vi "test Get-Set-Get Parameter Definitions.vi"(8 "error in":errorcluster, 11 "TestCase in":refnum<class "Scripting.lvclass">) -> (0 "error out":errorcluster, 3 "TestCase out":refnum<class "Scripting.lvclass">)   [LabVIEW 2020, in "Scripting.lvclass"]
uses:
  Scripting.lvclass
  Shared/Parameter Definition.ctl
  <vilib>/NI/NI VeriStand Encoding and Decoding/Encoding.ctl
  Shared/Direction.ctl
  Shared/SDI.ctl
  Shared/Transfer Type.ctl
  Scripting.lvclass/Scripting.ctl
  <vilib>/addons/_JKI Toolkits/VI Tester/TestCase.llb/TestCase.lvclass
  Scripting/AIM/AIM ARINC 429 Scripting.lvlib
  <vilib>/NI/NI VeriStand Encoding and Decoding/Encoding and Decoding.lvlib
  Shared/Transfer Speed.ctl
  C:/Program Files (x86)/National Instruments/LabVIEW 2020/vi.lib/addons/_JKI Toolkits/VI Tester/TestCase.llb/TestCase.lvclass
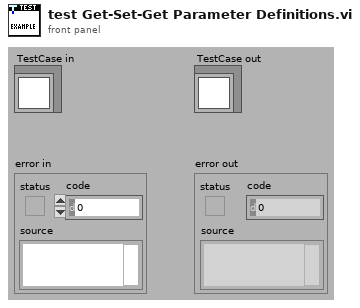
[diagram p1: front panel]
types:
  T1 = typedef "Transfer Speed.ctl" = enum16{"LO (12.5 kb/s)", "HI (100 kb/s)"}
  T2 = typedef "Transfer Type.ctl" = enum16{"Scheduled", "Acyclic", "Block", "Strobe"}
  T3 = typedef "Direction.ctl" = enum16{"Rx", "Tx"}
  T4 = typedef "SDI.ctl" = i32
  T5 = typedef "Parameter Definition.ctl" = cluster{"start index":i32, "size":i32, "encoding":T6, "signed":bool, "scale multiplier":dbl, "scale offset":dbl, "default value":dbl}
  T6 = typedef "Encoding and Decoding.lvlib/Encoding.ctl" = enum16{"BNR", "BCD", "Discrete"}
  T7 = typedef "Custom Device API.lvlib/Custom Device Item Ref.ctl" = u64
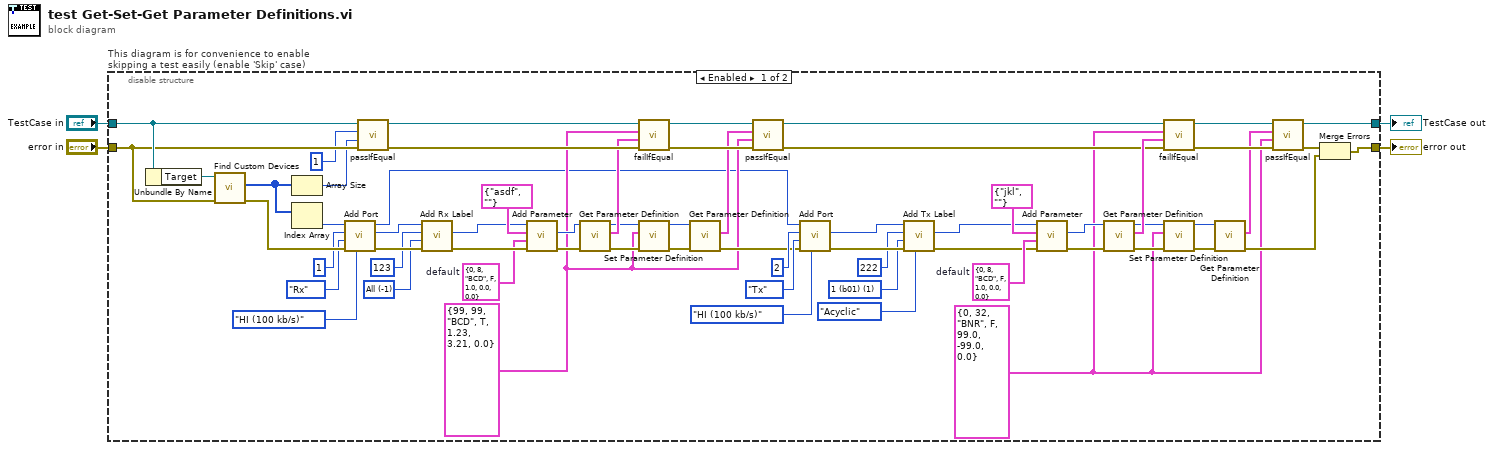
[diagram p0: block diagram]
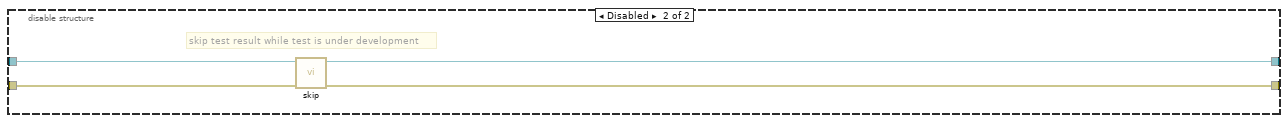
[diagram p2: hidden frame]
diagram:
  n1 = disable-structure "This diagram is for convenience to enable skipping a test easily (enable 'Skip' case)" shown="Enabled" {
    disable-tunnel: "TestCase in" -> [w66 w71]
    disable-tunnel: [w41 w69] -> w1
    disable-tunnel: [w60 w70] -> w3
    disable-tunnel: "error in" -> [w65 w68]
    frame Enabled {
      w11 = T4 1 items=["All"=-1, "0 (b00)"=0, "1 (b01)"=1, "2 (b10)"=2, "3 (b11)"=3] ("SDI value")
      w21 = T5 {"start index"=0, "size"=8, "encoding"=enum."BCD", "signed"=FALSE, "scale multiplier"=1.0, "scale offset"=0.0, "default value"=0.0}  # default
      w24 = T5 {"start index"=0, "size"=8, "encoding"=enum."BCD", "signed"=FALSE, "scale multiplier"=1.0, "scale offset"=0.0, "default value"=0.0}  # default
      w29 = T4 -1 items=["All"=-1, "0 (b00)"=0, "1 (b01)"=1, "2 (b10)"=2, "3 (b11)"=3] ("SDI value")
      w22 = T5 {"start index"=99, "size"=99, "encoding"=enum."BCD", "signed"=TRUE, "scale multiplier"=1.23, "scale offset"=3.21, "default value"=0.0} ("parameter definition")
      w15 = T5 {"start index"=0, "size"=32, "encoding"=enum."BNR", "signed"=FALSE, "scale multiplier"=99.0, "scale offset"=-99.0, "default value"=0.0} ("parameter definition")
      n2 = Unbundle By Name(w66) -> ("Target"=w67:refnum<k24>)
      n3 = call "Find Custom Devices.vi"("error in"=w65, "target in"=w67) -> ("error out"=w38:errorcluster, "AIM ARINC 429 custom devices"=w40:u64[])  [unwired: 7 in, 1 out]
      n4 = Array Size(array=w40) -> (size(s)=w63:i32)
      n5 = Index Array(array=w40) -> (element=w39:u64)  [unwired: 1 in]
      n6 = call "Add Port.vi"("speed"=Transfer_Speed."HI (100 kb/s)", "error in"=w38, "direction"=Direction."Rx", "port number"=u16 1, "AIM ARINC 429 custom device in"=w39) -> ("error out"=w31:errorcluster, "port"=w32:T7, "AIM ARINC 429 custom device out"=w10:T7)  [unwired: 4 in]
      n7 = call-dynamic "passIfEqual.vi"("error in (no error)"=w65, "y"=w63, "x"=1 ("size(s)"), "TestCase in"=w66) -> ("error out"=w61:errorcluster, "TestCase out"=w62:refnum<class "Scripting.lvclass">)  [unwired: 6 in]
      n8 = call "Add Rx Label.vi"("error in"=w31, "SDI value"=w29, "label value"=u32 123, "port in"=w32) -> ("error out"=w27:errorcluster, "label"=w8:T7)  [unwired: 5 in, 1 out]
      n9 = call "Add Parameter.vi"("error in"=w27, "parameter encoding"=w24, "parameter definition"=cluster{"name":string, "unit":string} {"name"="asdf", "unit"=""}, "label in"=w8) -> ("error out"=w25:errorcluster, "parameter"=w26:T7)  [unwired: 5 in, 1 out]
      n10 = call "Get Parameter Definition.vi"("error in"=w25, "parameter ref in"=w26) -> ("error out"=w57:errorcluster, "parameter definition"=w58:T5, "parameter ref out"=w56:T7)  [unwired: 7 in]
      n11 = call-dynamic "failIfEqual.vi"("error in (no error)"=w61, "y"=w58, "x"=w22, "TestCase in"=w62) -> ("error out"=w53:errorcluster, "TestCase out"=w52:refnum<class "Scripting.lvclass">)  [unwired: 6 in]
      n12 = call "Set Parameter Definition.vi"("error in"=w57, "parameter definition"=w22, "parameter ref in"=w56) -> ("error out"=w55:errorcluster, "parameter ref out"=w54:T7)  [unwired: 7 in]
      n13 = call "Get Parameter Definition.vi"("error in"=w55, "parameter ref in"=w54) -> ("error out"=w33:errorcluster, "parameter definition"=w23:T5)  [unwired: 7 in, 1 out]
      n14 = call-dynamic "passIfEqual.vi"("error in (no error)"=w53, "y"=w22, "x"=w23, "TestCase in"=w52) -> ("error out"=w51:errorcluster, "TestCase out"=w50:refnum<class "Scripting.lvclass">)  [unwired: 6 in]
      n15 = call "Add Port.vi"("speed"=Transfer_Speed."HI (100 kb/s)", "error in"=w33, "direction"=Direction."Tx", "port number"=u16 2, "AIM ARINC 429 custom device in"=w10) -> ("error out"=w19:errorcluster, "port"=w18:T7)  [unwired: 4 in, 1 out]
      n16 = call "Add Tx Label.vi"("transfer type"=Transfer_Type."Acyclic", "error in"=w19, "SDI value"=w11, "label value"=u32 222, "port in"=w18) -> ("error out"=w13:errorcluster, "label"=w7:T7)  [unwired: 4 in, 1 out]
      n17 = call "Add Parameter.vi"("error in"=w13, "parameter encoding"=w21, "parameter definition"=cluster{"name":string, "unit":string} {"name"="jkl", "unit"=""}, "label in"=w7) -> ("error out"=w17:errorcluster, "parameter"=w16:T7)  [unwired: 5 in, 1 out]
      n18 = call "Get Parameter Definition.vi"("error in"=w17, "parameter ref in"=w16) -> ("error out"=w47:errorcluster, "parameter definition"=w59:T5, "parameter ref out"=w46:T7)  [unwired: 7 in]
      n19 = call-dynamic "failIfEqual.vi"("error in (no error)"=w51, "y"=w59, "x"=w15, "TestCase in"=w50) -> ("error out"=w44:errorcluster, "TestCase out"=w42:refnum<class "Scripting.lvclass">)  [unwired: 6 in]
      n20 = call "Set Parameter Definition.vi"("error in"=w47, "parameter definition"=w15, "parameter ref in"=w46) -> ("error out"=w48:errorcluster, "parameter ref out"=w49:T7)  [unwired: 7 in]
      n21 = call "Get Parameter Definition.vi"("error in"=w48, "parameter ref in"=w49) -> ("error out"=w45:errorcluster, "parameter definition"=w14:T5)  [unwired: 7 in, 1 out]
      n22 = call-dynamic "passIfEqual.vi"("error in (no error)"=w44, "y"=w15, "x"=w14, "TestCase in"=w42) -> ("error out"=w43:errorcluster, "TestCase out"=w41:refnum<class "Scripting.lvclass">)  [unwired: 6 in]
      n23 = Merge Errors(w43, w45) -> (w60:errorcluster)
    }
    frame Disabled {
      # "skip test result while test is under development"
      n24 = call <vilib>:"skip.vi"("error in (no error)"=w68, "TestCase in"=w71) -> ("error out"=w70:errorcluster, "TestCase out"=w69:refnum<class "Scripting.lvclass">)  [unwired: 8 in]
    }
  }
  "error out" <- w3
  "TestCase out" <- w1
